vi "PackBoolean.vi"(10 "[booleans] as [U8]":u8[](array[numeric])) -> (1 "[packed (8) booleans] as [u8]":u8[](array[numeric]), 3 "Empty Color Table":u8[](array[numeric]))   [LabVIEW 2024]
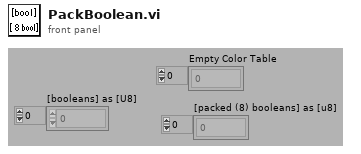
[diagram p1: front panel]
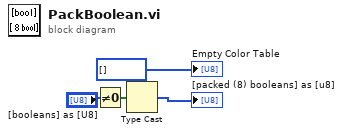
[diagram p0: block diagram]
diagram:
  w4 = u8[] [] ("initialized array")
  n1 = Not Equal To 0?(x="[booleans] as [U8]") -> (x != 0?=w3:bool[])
  n2 = Type Cast(type=w4, x=w3) -> (*(type *) &x=→"[packed (8) booleans] as [u8]":u8[])
  "Empty Color Table" <- w4
